vi "ep_Scaling Sensitivity (Single Line).vi"(8 "error in (no error)":errorcluster, 9 "system info in":refnum<class "EP System Info.lvclass">, 10 "sensitivity":dbl[](array[numeric]), 11 "waveforms in":waveform(dbl)[](array[waveform])) -> (0 "error out":errorcluster, 1 "system info out":refnum<class "EP System Info.lvclass">, 3 "waveforms out":waveform(dbl)[](array[waveform]))   [LabVIEW 2014, in "NI_EP_Power Quality.lvlib"]
uses:
  <vilib>/addons/Electrical Power/PQ/NI_EP_Power Quality.lvlib
  <vilib>/addons/Electrical Power/PQ/Common/Classes/System Info/EP System Info.lvclass
  <vilib>/addons/Electrical Power/PQ/Common/Controls/ep_AI Data Channel.ctl
  <vilib>/addons/Electrical Power/PQ/Scaling_Calibration/subVIs/ep_Compute Third Current (DBL WFM).vi
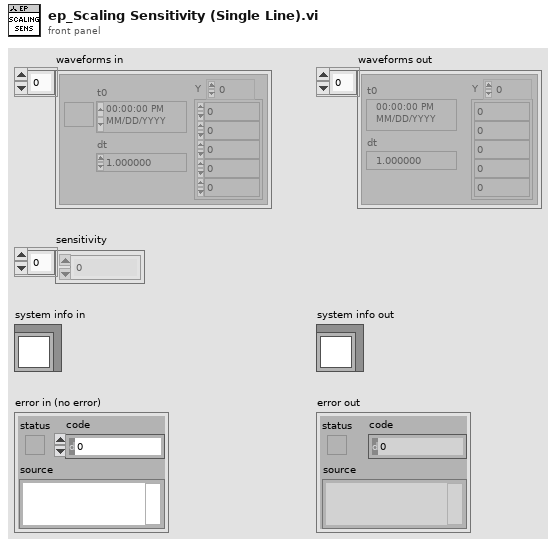
[diagram p1: front panel]
types:
  T1 = typedef "NI_EP_Power Quality.lvlib/ep_AI Data Channel.ctl" = enum16{"Voltage Phase A (L1)", "Voltage Phase B (L2)", "Voltage Phase C (L3)", "Voltage Phase N (Neutral)", "Current Phase A (L1)", "Current Phase B (L2)", "Current Phase C (L3)", "Current Phase N (Neutral)"}
  T2 = typedef "NI_EP_Power Quality.lvlib/ep_Wiring.ctl" = enum16{"4xUph + 4xI", "3xUph + 4xI", "3xUline + 4xI", "3xUph + 3xI", "3xUline + 3xI", "3xUph + 2xI", "3xUline + 2xI", "1xUph + 1xI"}
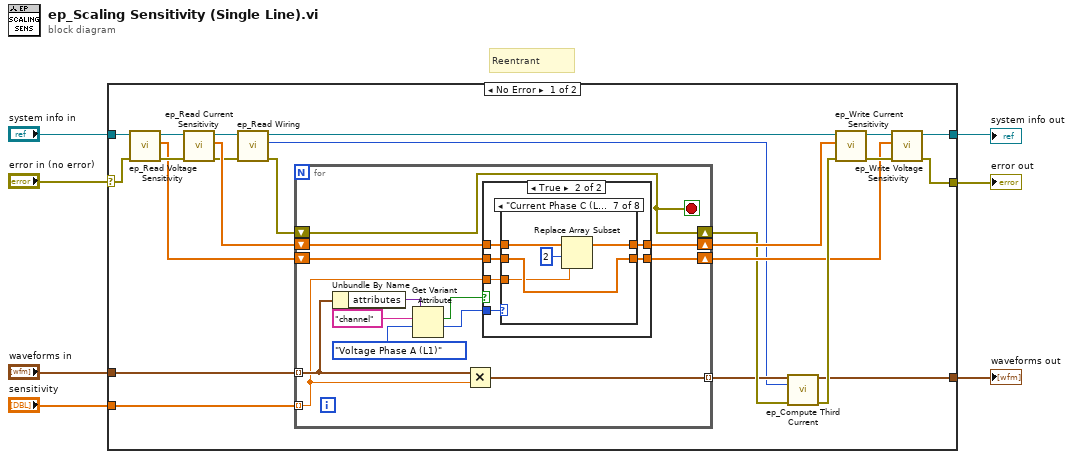
[diagram p0: block diagram]
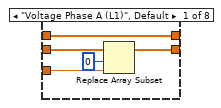
[diagram p3: hidden frame]
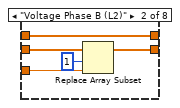
[diagram p4: hidden frame]
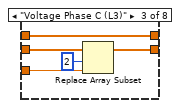
[diagram p5: hidden frame]
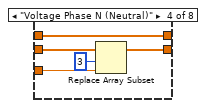
[diagram p6: hidden frame]
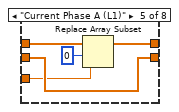
[diagram p7: hidden frame]
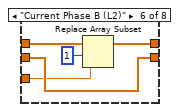
[diagram p8: hidden frame]
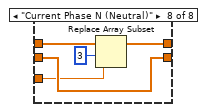
[diagram p9: hidden frame]
diagram:
  # "Reentrant"
  n1 = case shown="No Error" "error in (no error)" {
    selector: "error in (no error)" -> [w8 w93]
    tunnel: "system info in" -> [w18 w94]
    tunnel: "sensitivity" -> [w17 _]
    tunnel: "waveforms in" -> [w16 w92]
    tunnel: [w15 w94] -> w4
    tunnel: [w14 w93] -> w3
    tunnel: [w13 w92] -> w2
    frame No Error {
      n2 = call <vilib>:"ep_Read Voltage Sensitivity.vi"("error in (no error)"=w8, "system info in"=w18) -> ("error out"=w29:errorcluster, "voltage sensitivity"=w28:dbl[], "system info out"=w30:refnum<class "EP System Info.lvclass">)  [unwired: 7 in]
      n3 = call <vilib>:"ep_Read Current Sensitivity.vi"("error in (no error)"=w29, "system info in"=w30) -> ("error out"=w19:errorcluster, "current sensitivity"=w27:dbl[], "system info out"=w21:refnum<class "EP System Info.lvclass">)  [unwired: 7 in]
      n4 = call <vilib>:"ep_Read Wiring.vi"("error in (no error)"=w19, "system info in"=w21) -> ("error out"=w12:errorcluster, "wiring"=w9:T2, "system info out"=w20:refnum<class "EP System Info.lvclass">)  [unwired: 6 in, 1 out]
      n5 = for {
        tunnel: w16 -> [w40] mode=indexing
        tunnel: w17 -> [w35] mode=indexing
        tunnel: [w43] -> w10 mode=indexing
        shift-right: [w37] -> w24
        shift-left: w27 -> [w39]
        shift-right: [w36] -> w22
        shift-left: w28 -> [w38]
        shift-right: [w31] -> w11
        shift-left: w12 -> [w31]
        stop <- w31 stop-if-true
        n6 = Unbundle By Name(w40) -> ("attributes"=w42:variant)
        n7 = Get Variant Attribute(Variant=w42, name="channel", default value (empty Variant)=ep_AI_Data_Channel."Voltage Phase A (L1)" ("AI data channel")) -> (found=w34:bool, value=w33:T1)  [unwired: 1 in, 2 out]
        n8 = Multiply(x=w40, y=w35) -> (x*y=w43:waveform(dbl))
        n9 = case shown="True" w34 {
          tunnel: w33 -> [_ w51]
          tunnel: w35 -> [_ w50]
          tunnel: w38 -> [w45 w49]
          tunnel: [w45 w46] -> w36
          tunnel: [w44 w48] -> w37
          tunnel: w39 -> [w44 w47]
          frame False {
          }
          frame True {
            n10 = case shown="\"Current Phase C (L3)\"" w51 {
              tunnel: w50 -> [w55 w60 w65 w70 w72 w77 w82 w87]
              tunnel: w49 -> [w56 w61 w66 w71 w73 w78 w83 w88]
              tunnel: [w54 w59 w64 w69 w74 w79 w84 w89] -> w48
              tunnel: w47 -> [w54 w59 w64 w69 w75 w80 w85 w90]
              tunnel: [w53 w58 w63 w68 w73 w78 w83 w88] -> w46
              frame "Voltage Phase A (L1)", Default {
                n11 = Replace Array Subset(array=w56, new element=w55, index=0) -> (w53:dbl[])
              }
              frame "Voltage Phase B (L2)" {
                n12 = Replace Array Subset(array=w61, new element=w60, index=1) -> (w58:dbl[])
              }
              frame "Voltage Phase C (L3)" {
                n13 = Replace Array Subset(array=w66, new element=w65, index=2) -> (w63:dbl[])
              }
              frame "Voltage Phase N (Neutral)" {
                n14 = Replace Array Subset(array=w71, new element=w70, index=3) -> (w68:dbl[])
              }
              frame "Current Phase A (L1)" {
                n15 = Replace Array Subset(array=w75, new element=w72, index=0) -> (w74:dbl[])
              }
              frame "Current Phase B (L2)" {
                n16 = Replace Array Subset(array=w80, new element=w77, index=1) -> (w79:dbl[])
              }
              frame "Current Phase C (L3)" {
                n17 = Replace Array Subset(array=w85, new element=w82, index=2) -> (w84:dbl[])
              }
              frame "Current Phase N (Neutral)" {
                n18 = Replace Array Subset(array=w90, new element=w87, index=3) -> (w89:dbl[])
              }
            }
          }
        }
      }
      n19 = call-poly <vilib>:"ep_Compute Third Current.vi"("current waveforms in"=w10, "wiring"=w9, "error in (no error)"=w11) -> ("current waveforms out"=w13:waveform(dbl)[], "error out"=w23:errorcluster)  [unwired: 11 in]
      n20 = call <vilib>:"ep_Write Current Sensitivity.vi"("error in (no error)"=w23, "current sensitivity"=w24, "system info in"=w20) -> ("error out"=w26:errorcluster, "system info out"=w25:refnum<class "EP System Info.lvclass">)  [unwired: 7 in]
      n21 = call <vilib>:"ep_Write Voltage Sensitivity.vi"("error in (no error)"=w26, "voltage sensitivity"=w22, "system info in"=w25) -> ("error out"=w14:errorcluster, "system info out"=w15:refnum<class "EP System Info.lvclass">)  [unwired: 7 in]
    }
    frame Error {
    }
  }
  "waveforms out" <- w2
  "error out" <- w3
  "system info out" <- w4
